vi "LEDC SWIR 2936 Init.vi"(0 "LEDAD Port":refnum<visa-resource-name>="COM7", 1 "Wavelength":string, 5 "Light Meter Port":refnum<visa-resource-name>="COM4", 11 "error in (no error)":errorcluster, 12 "Channel":enum16{"Chn1", "Chn2"}(ring)) -> (3 "In Progress":bool, 4 "LEDAD Port out":refnum<visa-resource-name>, 6 "Light Meter Port out":refnum<visa-resource-name>, 14 "Done":bool, 15 "error out":errorcluster)   [LabVIEW 2010]
panel:
  # "nm"
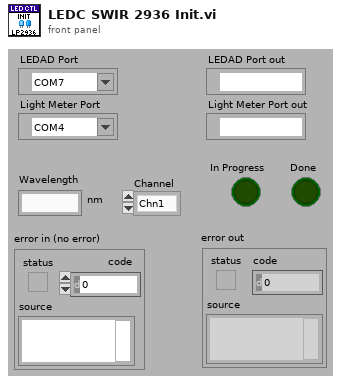
[diagram p1: front panel]
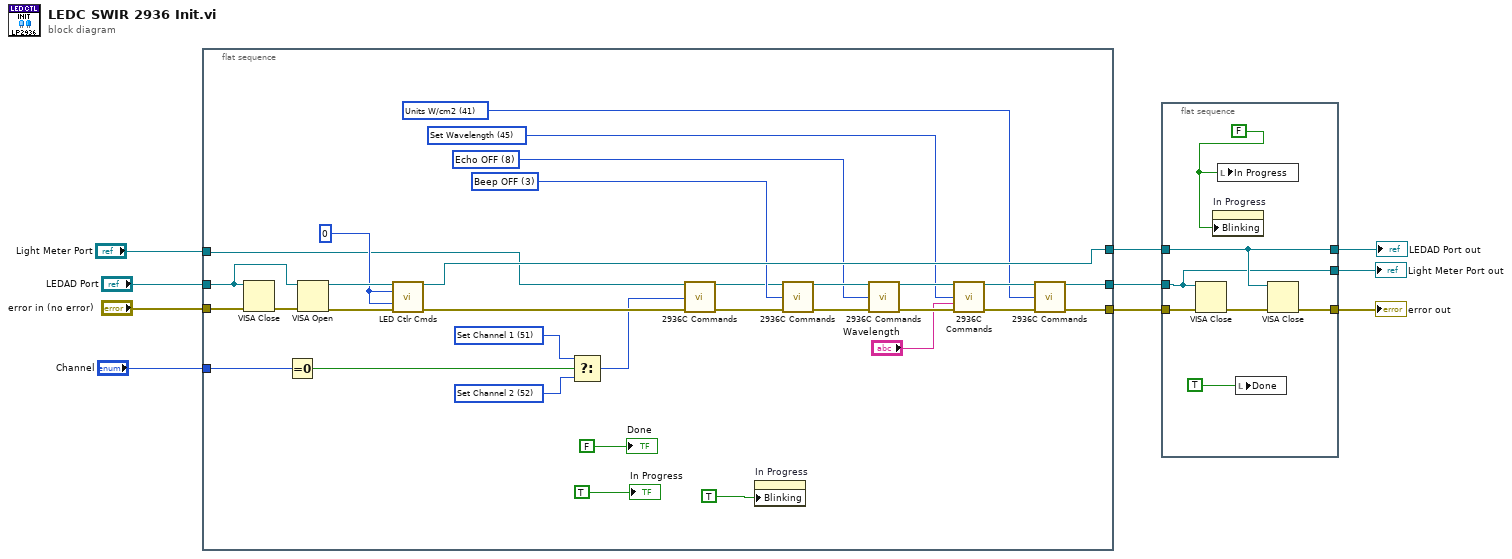
[diagram p0: block diagram]
diagram:
  n1 = flat-sequence {
    tunnel: "error in (no error)" -> [w42]
    tunnel: "LEDAD Port" -> [w40]
    tunnel: "Light Meter Port" -> [w18]
    tunnel: [w31] -> w3
    tunnel: [w30] -> w4
    tunnel: [w27] -> w2
    tunnel: "Channel" -> [w15]
    frame #0 {
      w13 = u16 52 items=["Attenuator OFF", "Attenuator ON", "Attenuator Query", "Beep OFF", "Beep ON", "Beep Query", "Clear Status Reg", "Get Power (nW)", "Echo OFF", "Echo ON", "Echo Query", "No Filter", "Analog Filter", "Digital FIlter", "Filter Query", "Hold", "Go", "Go Query", "Backlight OFF", "Backlight Medium", "Backlight High", "Backlight Query", "Set Dsplay Screen 0", "Set Display Screen 1", "Display Screen Query", "Mode DC Continuous", "Mode DC Single", "Mode Integrate", "Identification", "Auto Range", "Auto Range Query", "Signal Range 0", "Signal Range 1", "Signal Range 2", "Signal Range 3", "Signal Range 4", "Signal Range 5", "Signal Range 6", "Signal Range Query", "Store Reference", "Units W", "Units W/cm2", "Units dBm", "Units Joules", "Units Query", "Set Wavelength", "Wavelength Querry", "Mode Pesk-to-Peak Cont.", "Mode Peak-to-Peak Sing.", "Mode Query", "Channel Querry", "Set Channel 1", "Set Channel 2"] ("Command")
      w14 = u16 51 items=["Attenuator OFF", "Attenuator ON", "Attenuator Query", "Beep OFF", "Beep ON", "Beep Query", "Clear Status Reg", "Get Power (nW)", "Echo OFF", "Echo ON", "Echo Query", "No Filter", "Analog Filter", "Digital FIlter", "Filter Query", "Hold", "Go", "Go Query", "Backlight OFF", "Backlight Medium", "Backlight High", "Backlight Query", "Set Dsplay Screen 0", "Set Display Screen 1", "Display Screen Query", "Mode DC Continuous", "Mode DC Single", "Mode Integrate", "Identification", "Auto Range", "Auto Range Query", "Signal Range 0", "Signal Range 1", "Signal Range 2", "Signal Range 3", "Signal Range 4", "Signal Range 5", "Signal Range 6", "Signal Range Query", "Store Reference", "Units W", "Units W/cm2", "Units dBm", "Units Joules", "Units Query", "Set Wavelength", "Wavelength Querry", "Mode Pesk-to-Peak Cont.", "Mode Peak-to-Peak Sing.", "Mode Query", "Channel Querry", "Set Channel 1", "Set Channel 2"] ("Command")
      w20 = u16 41 items=["Attenuator OFF", "Attenuator ON", "Attenuator Query", "Beep OFF", "Beep ON", "Beep Query", "Clear Status Reg", "Get Power (nW)", "Echo OFF", "Echo ON", "Echo Query", "No Filter", "Analog Filter", "Digital FIlter", "Filter Query", "Hold", "Go", "Go Query", "Backlight OFF", "Backlight Medium", "Backlight High", "Backlight Query", "Set Dsplay Screen 0", "Set Display Screen 1", "Display Screen Query", "Mode DC Continuous", "Mode DC Single", "Mode Integrate", "Identification", "Auto Range", "Auto Range Query", "Signal Range 0", "Signal Range 1", "Signal Range 2", "Signal Range 3", "Signal Range 4", "Signal Range 5", "Signal Range 6", "Signal Range Query", "Store Reference", "Units W", "Units W/cm2", "Units dBm", "Units Joules", "Units Query", "Set Wavelength", "Wavelength Querry", "Mode Pesk-to-Peak Cont.", "Mode Peak-to-Peak Sing.", "Mode Query", "Channel Querry", "Set Channel 1", "Set Channel 2"] ("Command")
      w21 = u16 45 items=["Attenuator OFF", "Attenuator ON", "Attenuator Query", "Beep OFF", "Beep ON", "Beep Query", "Clear Status Reg", "Get Power (nW)", "Echo OFF", "Echo ON", "Echo Query", "No Filter", "Analog Filter", "Digital FIlter", "Filter Query", "Hold", "Go", "Go Query", "Backlight OFF", "Backlight Medium", "Backlight High", "Backlight Query", "Set Dsplay Screen 0", "Set Display Screen 1", "Display Screen Query", "Mode DC Continuous", "Mode DC Single", "Mode Integrate", "Identification", "Auto Range", "Auto Range Query", "Signal Range 0", "Signal Range 1", "Signal Range 2", "Signal Range 3", "Signal Range 4", "Signal Range 5", "Signal Range 6", "Signal Range Query", "Store Reference", "Units W", "Units W/cm2", "Units dBm", "Units Joules", "Units Query", "Set Wavelength", "Wavelength Querry", "Mode Pesk-to-Peak Cont.", "Mode Peak-to-Peak Sing.", "Mode Query", "Channel Querry", "Set Channel 1", "Set Channel 2"] ("Command")
      w22 = u16 8 items=["Attenuator OFF", "Attenuator ON", "Attenuator Query", "Beep OFF", "Beep ON", "Beep Query", "Clear Status Reg", "Get Power (nW)", "Echo OFF", "Echo ON", "Echo Query", "No Filter", "Analog Filter", "Digital FIlter", "Filter Query", "Hold", "Go", "Go Query", "Backlight OFF", "Backlight Medium", "Backlight High", "Backlight Query", "Set Dsplay Screen 0", "Set Display Screen 1", "Display Screen Query", "Mode DC Continuous", "Mode DC Single", "Mode Integrate", "Identification", "Auto Range", "Auto Range Query", "Signal Range 0", "Signal Range 1", "Signal Range 2", "Signal Range 3", "Signal Range 4", "Signal Range 5", "Signal Range 6", "Signal Range Query", "Store Reference", "Units W", "Units W/cm2", "Units dBm", "Units Joules", "Units Query", "Set Wavelength", "Wavelength Querry", "Mode Pesk-to-Peak Cont.", "Mode Peak-to-Peak Sing.", "Mode Query", "Channel Querry", "Set Channel 1", "Set Channel 2"] ("Command")
      w23 = u16 3 items=["Attenuator OFF", "Attenuator ON", "Attenuator Query", "Beep OFF", "Beep ON", "Beep Query", "Clear Status Reg", "Get Power (nW)", "Echo OFF", "Echo ON", "Echo Query", "No Filter", "Analog Filter", "Digital FIlter", "Filter Query", "Hold", "Go", "Go Query", "Backlight OFF", "Backlight Medium", "Backlight High", "Backlight Query", "Set Dsplay Screen 0", "Set Display Screen 1", "Display Screen Query", "Mode DC Continuous", "Mode DC Single", "Mode Integrate", "Identification", "Auto Range", "Auto Range Query", "Signal Range 0", "Signal Range 1", "Signal Range 2", "Signal Range 3", "Signal Range 4", "Signal Range 5", "Signal Range 6", "Signal Range Query", "Store Reference", "Units W", "Units W/cm2", "Units dBm", "Units Joules", "Units Query", "Set Wavelength", "Wavelength Querry", "Mode Pesk-to-Peak Cont.", "Mode Peak-to-Peak Sing.", "Mode Query", "Channel Querry", "Set Channel 1", "Set Channel 2"] ("Command")
      w26 = 0
      n2 = VISA Close(VISA resource name=w40, error in (no error)=w42) -> (error out=w41:errorcluster)
      n3 = Equal To 0?(x=w15) -> (x = 0?=w12:bool)
      n4 = VISA Open(error in (no error)=w41, VISA resource name=w40) -> (VISA resource name=w29:refnum<visa-resource-name>, error out=w28:errorcluster)  [unwired: 3 in]
      n5 = call "LED Ctlr Cmds.vi"("VISA session"=w29, "Intensity"=w26, "Enable"=w26, "error in (no error)"=w28) -> ("VISA session out"=w27:refnum<visa-resource-name>, "error out"=w19:errorcluster)  [unwired: 7 in, 3 out]
      n6 = Select(t=w14, s=w12, f=w13) -> (s? t:f=w11:u16)
      n7 = call "2936C Commands.vi"("Instrument Resource Name"=w18, "Command"=w11, "error in (no error)"=w19) -> ("VISA resource name out"=w17:refnum<visa-resource-name>, "error out"=w16:errorcluster)  [unwired: 8 in, 3 out]
      n8 = property on="In Progress" class="Bool (strict)"("Blinking"=TRUE) -> ()  [unwired: 2 in, 2 out]
      n9 = call "2936C Commands.vi"("Instrument Resource Name"=w17, "Command"=w23, "error in (no error)"=w16) -> ("VISA resource name out"=w25:refnum<visa-resource-name>, "error out"=w24:errorcluster)  [unwired: 8 in, 3 out]
      n10 = call "2936C Commands.vi"("Instrument Resource Name"=w25, "Command"=w22, "error in (no error)"=w24) -> ("VISA resource name out"=w38:refnum<visa-resource-name>, "error out"=w39:errorcluster)  [unwired: 8 in, 3 out]
      n11 = call "2936C Commands.vi"("Instrument Resource Name"=w38, "Command"=w21, "Wavelength"="Wavelength", "error in (no error)"=w39) -> ("VISA resource name out"=w33:refnum<visa-resource-name>, "error out"=w34:errorcluster)  [unwired: 7 in, 3 out]
      n12 = call "2936C Commands.vi"("Instrument Resource Name"=w33, "Command"=w20, "error in (no error)"=w34) -> ("VISA resource name out"=w31:refnum<visa-resource-name>, "error out"=w30:errorcluster)  [unwired: 8 in, 3 out]
      "Done" <- FALSE
      "In Progress" <- TRUE
    }
  }
  n13 = flat-sequence {
    tunnel: w3 -> [w45]
    tunnel: w4 -> [w47]
    tunnel: [w46] -> w5
    tunnel: w2 -> [w46]
    tunnel: [w45] -> w6
    tunnel: [w43] -> w7
    frame #0 {
      w49 = FALSE
      n14 = VISA Close(VISA resource name=w45, error in (no error)=w47) -> (error out=w44:errorcluster)
      n15 = property on="In Progress" class="Bool (strict)"("Blinking"=w49) -> ()  [unwired: 2 in, 2 out]
      n16 = local write "In Progress"(w49) -> ()
      n17 = local write "Done"(TRUE) -> ()
      n18 = VISA Close(VISA resource name=w46, error in (no error)=w44) -> (error out=w43:errorcluster)
    }
  }
  "LEDAD Port out" <- w5
  "Light Meter Port out" <- w6
  "error out" <- w7
